vi "ueye error handling.vi"(4 "Error Code":i32, 6 "reference in":refnum<k24>, 9 "Error In":errorcluster) -> (1 "Error Out":errorcluster)   [LabVIEW 2022 SP3, in "Vision.lvlib"]
uses:
  Vision.lvlib
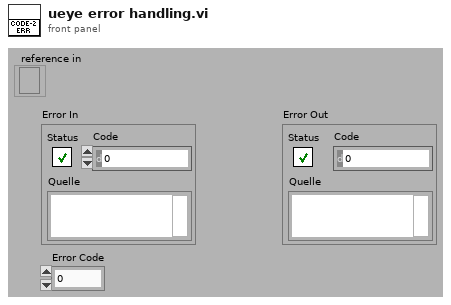
[diagram p1: front panel]
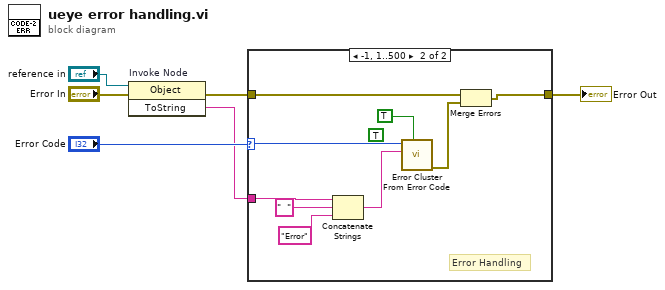
[diagram p0: block diagram]
diagram:
  n1 = invoke on="Invoke Node" class="Object" method="ToString"(reference="reference in", error in="Error In") -> (error out=w3:errorcluster, "ToString"=w2:string)  [unwired: 1 in, 1 out]
  n2 = case shown="-1, 1..500" "Error Code" {
    selector: "Error Code" -> [_ w11]
    tunnel: w3 -> [w7 w13]
    tunnel: [w7 w12] -> w6
    tunnel: w2 -> [_ w14]
    frame 0, Default {
    }
    frame -1, 1..500 {
      (unwired) TRUE
      # "Error Handling"
      n3 = Concatenate Strings(w14, "  ", "Error") -> (w10:string)
      n4 = call <vilib>:"Error Cluster From Error Code.vi"("show call chain? (False)"=TRUE, "error message (\"\")"=w10, "error code (0)"=w11) -> ("error out"=w9:errorcluster)  [unwired: 6 in]
      n5 = Merge Errors(w13, w9) -> (w12:errorcluster)
    }
  }
  "Error Out" <- w6
